vi "cluster.vi"() -> ()   [LabVIEW 2021]
panel:
  out "Name Cluster":cluster{"Course ID":string, "Department":string}
  out "Indicator Cluster":T1
  in  "Control Cluster":T1
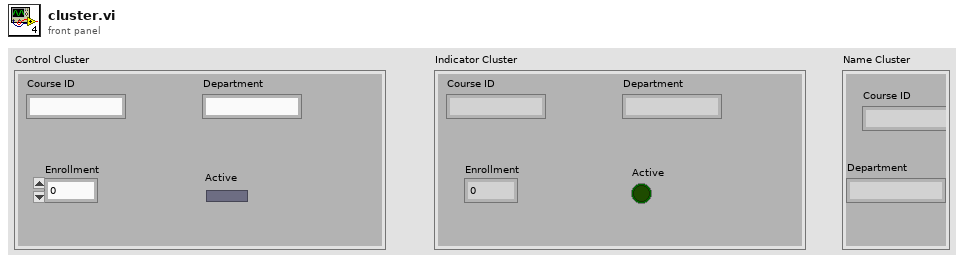
[diagram p1: front panel]
types:
  T1 = cluster{"Course ID":string, "Department":string, "Enrollment":dbl, "Active":bool}
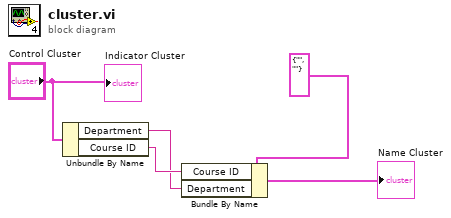
[diagram p0: block diagram]
diagram:
  n1 = Unbundle By Name("Control Cluster") -> ("Department"=w1:string, "Course ID"=w2:string)
  n2 = Bundle By Name(cluster=cluster{"Course ID":string, "Department":string} {"Course ID"="", "Department"=""} ("Name Cluster"), "Course ID"=w2, "Department"=w1) -> (→"Name Cluster":cluster{"Course ID":string, "Department":string})
  "Indicator Cluster" <- "Control Cluster"
